vi "Load File Data.vi"(10 "Path":path) -> (1 "Auto Data":dbl[][](array[numeric]))   [LabVIEW 2017]
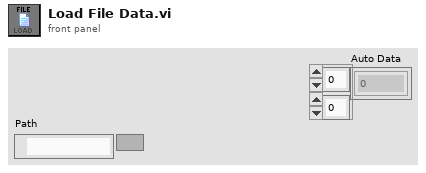
[diagram p1: front panel]
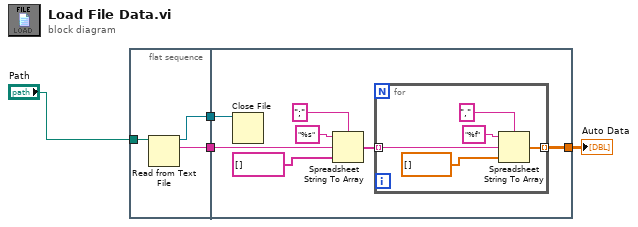
[diagram p0: block diagram]
diagram:
  n1 = flat-sequence {
    tunnel: "Path" -> [w7]
    tunnel: [w6] -> w4
    tunnel: [w5] -> w3
    tunnel: w4 -> [w10]
    tunnel: w3 -> [w9]
    tunnel: [w8] -> w1
    frame #0 {
      n2 = Read from Text File(file (use dialog)=w7) -> (refnum out=w6:refnum<file>, text=w5:string)  [unwired: 3 in, 2 out]
    }
    frame #1 {
      n3 = Close File(refnum=w10) -> ()  [unwired: 1 in, 2 out]
      n4 = Spreadsheet String To Array(delimiter (Tab)=";", format string="%s", spreadsheet string=w9, array type (2D Dbl)=string[] []) -> (array=w12:string[])
      n5 = for {
        tunnel: w12 -> [w19] mode=indexing
        tunnel: [w16] -> w8 mode=indexing
        n6 = Spreadsheet String To Array(delimiter (Tab)=",", format string="%f", spreadsheet string=w19, array type (2D Dbl)=dbl[] []) -> (array=w16:dbl[])
      }
    }
  }
  "Auto Data" <- w1
